vi "FrontLabel.vi"(11 "label":string) -> (3 "String":string)   [LabVIEW 2014, in "OPCUA XML.lvlib"]
uses:
  OPCUA XML.lvlib
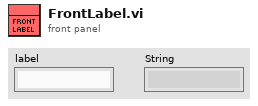
[diagram p1: front panel]
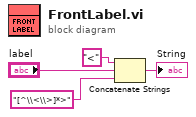
[diagram p0: block diagram]
diagram:
  n1 = Concatenate Strings("<" ("regular expression"), "label", "[^\\<\\>]*>" ("regular expression")) -> (→"String":string)
